vi "Create.vi"(8 "error in (no error)":errorcluster, 9 "Calculation Period (ms)":u32=500, 10 "XNET Session":refnum<k21>, 11 "CANBus_Load_Calculator in":refnum<class "CANBus_Load_Calculator.lvclass">) -> (0 "error out":errorcluster, 3 "CANBus_Load_Calculator out":refnum<class "CANBus_Load_Calculator.lvclass">)   [LabVIEW 2019, in "XNET-Bus-Load-Calculator.lvlib" / "CANBus_Load_Calculator.lvclass"]
uses:
  CANBus_Load_Calculator.lvclass
  GenBus/GenBus_Load_Calculator.lvclass
  <resource>/objmgr/xnet.rc
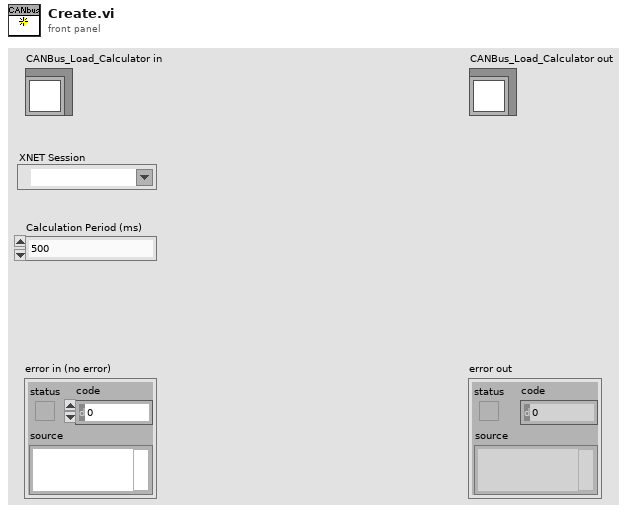
[diagram p1: front panel]
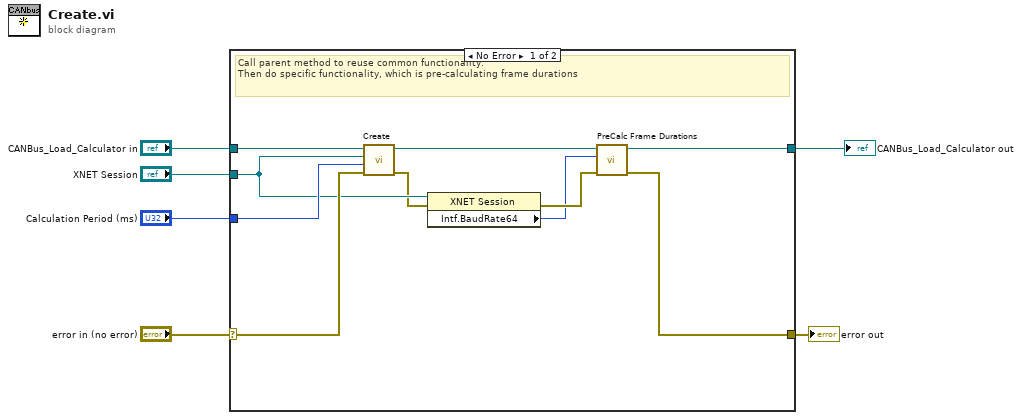
[diagram p0: block diagram]
diagram:
  n1 = case shown="No Error" "error in (no error)" {
    selector: "error in (no error)" -> [w14 w17]
    tunnel: [w12 w18] -> w6
    tunnel: "Calculation Period (ms)" -> [w16 _]
    tunnel: "XNET Session" -> [w11 _]
    tunnel: "CANBus_Load_Calculator in" -> [w15 w18]
    tunnel: [w7 w17] -> w1
    frame No Error {
      # "Call parent method to reuse common functionality.\nThen do specific functionality, which is pre-calculating frame durations"
      n2 = call-parent "Create.vi"("error in (no error)"=w14, "Calculation Period (ms)"=w16, "XNET Session"=w11, "GenBus_Load_Calculator in"=w15) -> ("error out"=w10:errorcluster, "GenBus_Load_Calculator out"=w13:refnum<class "CANBus_Load_Calculator.lvclass">)  [unwired: 6 in]
      n3 = property class="XNET Session"(reference=w11, error in=w10) -> (error out=w9:errorcluster, "Intf.BaudRate64"=w8:u64)  [unwired: 1 out]
      n4 = call "PreCalc Frame Durations.vi"("error in (no error)"=w9, "Baud Rate"=w8, "CAN Bus Class In"=w13) -> ("error out"=w7:errorcluster, "CAN Bus Class Out"=w12:refnum<class "CANBus_Load_Calculator.lvclass">)  [unwired: 7 in]
    }
    frame Error {
    }
  }
  "error out" <- w1
  "CANBus_Load_Calculator out" <- w6
